vi "Stability length measurement.vi"() -> ()   [LabVIEW 2018]
uses:
  <vilib>/DAQmx/write.llb/DAQmx Write (Analog DBL 1Chan 1Samp).vi
  <vilib>/DAQmx/read.llb/DAQmx Read (Analog DBL 1Chan 1Samp).vi
  <vilib>/DAQmx/create/channels.llb/DAQmx Create Channel (AO-Voltage-Basic).vi
  <vilib>/DAQmx/create/channels.llb/DAQmx Create Channel (AI-Voltage-Basic).vi
  <vilib>/DAQmx/miscellaneous.llb/DAQmx Fill In Error Info.vi
panel:
  in  "reignition channel":tag
  in  "stop":bool
  out "stable voltage":dbl
  out "steady state voltage":dbl
  in  "diode channel":tag
  in  "rf gen channel":tag
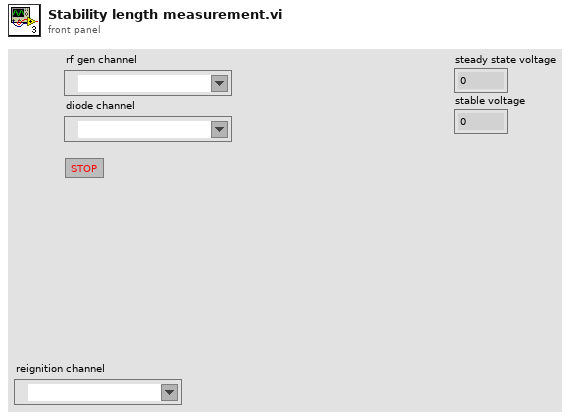
[diagram p1: front panel]
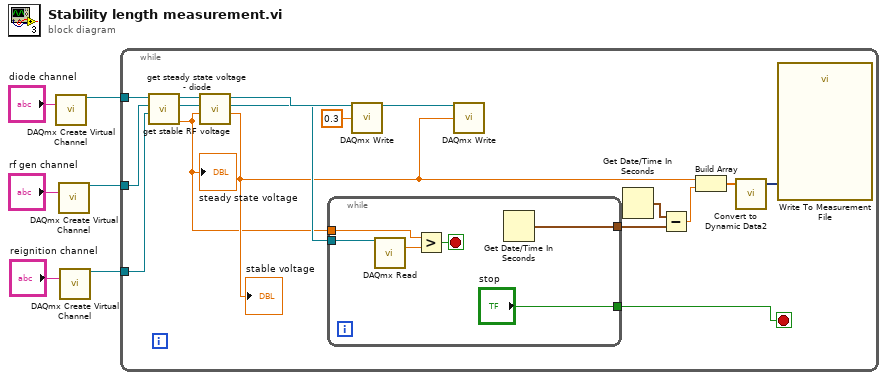
[diagram p0: block diagram]
diagram:
  n1 = call-poly <vilib>:"DAQmx Create Virtual Channel.vi"("physical channels"="diode channel") -> ("task out"=w3:refnum<k21>)  [unwired: 13 in, 1 out]
  n2 = call-poly <vilib>:"DAQmx Create Virtual Channel.vi"("physical channels"="rf gen channel") -> ("task out"=w4:refnum<k21>)  [unwired: 13 in, 1 out]
  n3 = call-poly <vilib>:"DAQmx Create Virtual Channel.vi"("physical channels"="reignition channel") -> ("task out"=w1:refnum<k21>)  [unwired: 13 in, 1 out]
  n4 = while {
    tunnel: w4 -> [w20]
    tunnel: w3 -> [w19]
    tunnel: w1 -> [w9]
    stop <- w11 stop-if-true
    n5 = call "get steady state voltage - diode.vi"("Reignition Task In"=w9, "Diode Task In"=w20, "RF Generator Task In"=w19) -> ("Output"=w10:dbl, "diode task out"=w7:refnum<k21>, "rf generator task out"=w8:refnum<k21>)  [unwired: 5 in, 1 out]
    "steady state voltage" <- w10
    n6 = call "get stable RF voltage.vi"("diode steady state voltage"=w10, "polarimeter task in"=w7, "rf gen task in"=w8) -> ("stable voltage"=w15:dbl, "polarimeter task out"=w18:refnum<k21>, "rf gen task out"=w23:refnum<k21>)  [unwired: 6 in]
    "stable voltage" <- w15
    n7 = while {
      tunnel: w18 -> [w29]
      tunnel: w10 -> [w27]
      tunnel: [w25] -> w16
      tunnel: ["stop"] -> w11
      stop <- w26 stop-if-true
      n8 = call-poly <vilib>:"DAQmx Read.vi"("task/channels in"=w29) -> ("data"=w28:dbl)  [unwired: 12 in, 2 out]
      n9 = Greater?(x=w27, y=w28) -> (0:w26:bool)
      n10 = Get Date/Time In Seconds() -> (seconds since 1Jan1904=w25:timestamp)
    }
    n11 = call-poly <vilib>:"DAQmx Write.vi"("task/channels in"=w23, "data"=0.3) -> ("task out"=w22:refnum<k21>)  [unwired: 11 in, 2 out]
    n12 = call-poly <vilib>:"DAQmx Write.vi"("task/channels in"=w22, "data"=w15) -> ()  [unwired: 11 in, 3 out]
    n13 = Get Date/Time In Seconds() -> (seconds since 1Jan1904=w17:timestamp)
    n14 = Subtract(x=w17, y=w16) -> (x-y=w14:dbl)
    n15 = Build Array(w15, w14) -> (w13:dbl[])
    n16 = call "Convert to Dynamic Data2"("Array"=w13) -> ("Dynamic Data Type"=w12:dynamicdata)  [unwired: 3 in]
    n17 = call "Write To Measurement File"("Signals"=w12) -> ()  [unwired: 16 in, 3 out]
  }
